vi "DT_Merge_Init.vi"(5 "right subset":cluster{"start idx":i32, "length":i32}, 7 "left subset":cluster{"start idx":i32, "length":i32}, 10 "Triangles In":i32[][](array[numeric]), 11 "Points In":cluster{"x":dbl, "y":dbl, "index":i32}[](array[cluster])) -> (0 "error":i32, 1 "Data":T1, 2 "Triangles Out":i32[][](array[numeric]), 3 "Points Out":cluster{"x":dbl, "y":dbl, "index":i32}[](array[cluster]))   [LabVIEW 2020, in "NI_AAL_Geometry.lvlib"]
uses:
  <vilib>/Analysis/NI_AAL_Geometry.lvlib
  <vilib>/Analysis/geometry.llb/DT_Merge_Find Next Triangulation_Data.ctl
  <vilib>/Analysis/geometry.llb/DT_Triangle Manager_Get Oppo Point_in Ghost.vi
  <vilib>/Analysis/geometry.llb/DT_Triangle Manager_Get Global Point Index.vi
  <vilib>/Analysis/geometry.llb/DT_Triangle Manager_Get Adj_by Edge.vi
  <vilib>/Analysis/geometry.llb/DT_Triangle Manager_Get Oppo Point.vi
  <vilib>/Analysis/geometry.llb/DT_Triangle Manager_Get Ghost Point.vi
  <vilib>/Analysis/geometry.llb/DT_Triangle Manager_Get Adj_by Point.vi
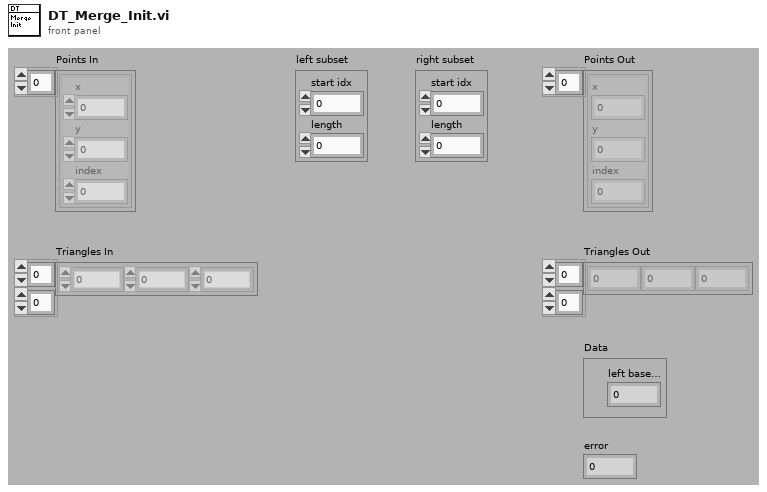
[diagram p1: front panel]
types:
  T1 = typedef "NI_AAL_Geometry.lvlib/DT_Merge_Find Next Triangulation_Data.ctl" = cluster{"left base point":i32, "left triangle":i32, "left local idx":i32, "right base point":i32, "right triangle":i32, "right local idx":i32, "Left Candidate Triangles":i32[], "Left Candidate Point Idx":i32[], "Right Candidate Triangles":i32[], "Right Candidate Point Idx":i32[], "cur triangle":i32}
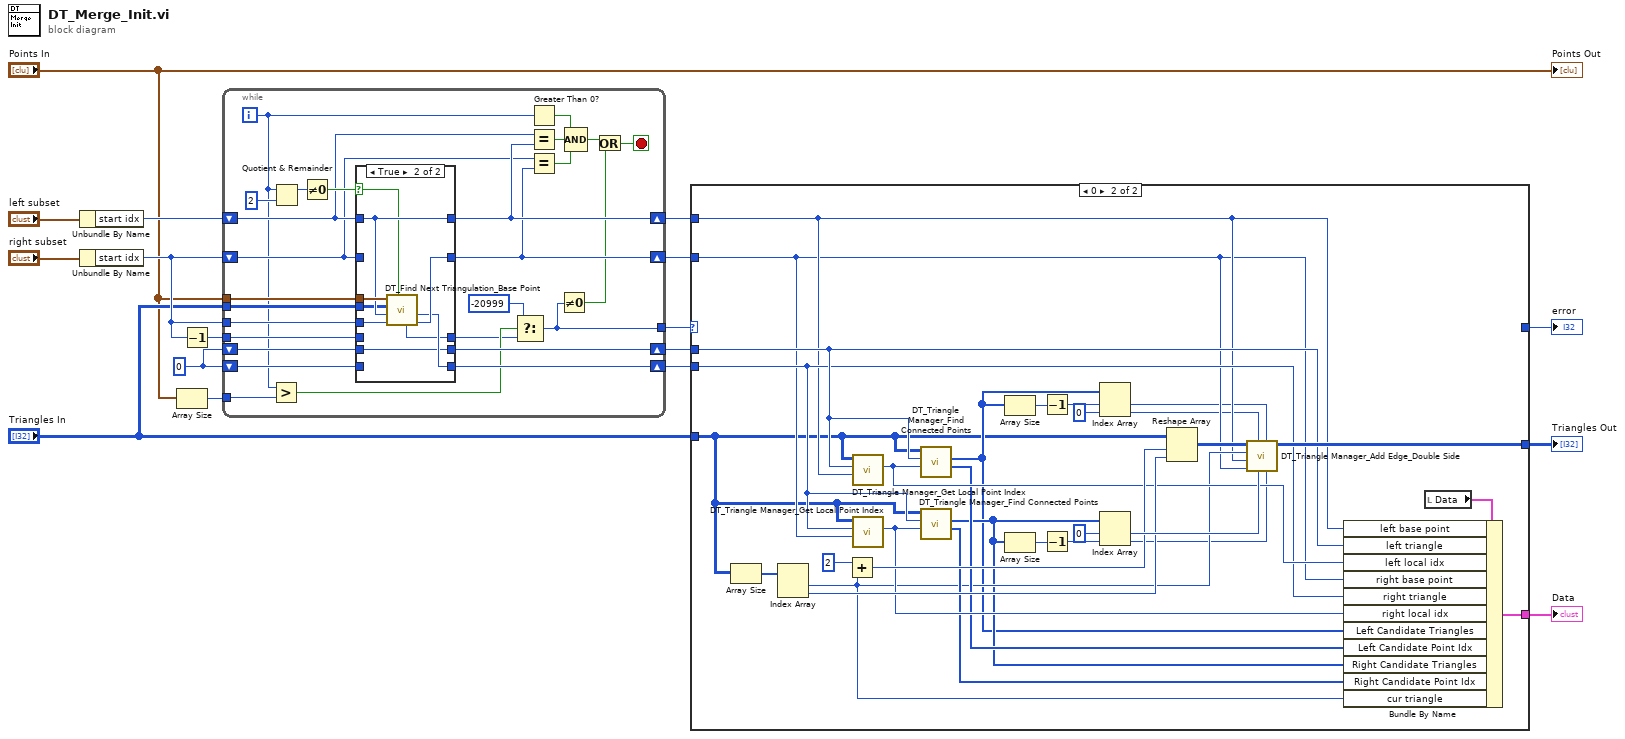
[diagram p0: block diagram]
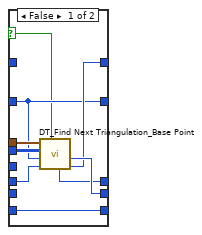
[diagram p3: hidden frame]
diagram:
  w15 = 0 ("triangle")
  n1 = Unbundle By Name("left subset") -> ("start idx"=w7:i32)
  n2 = Unbundle By Name("right subset") -> ("start idx"=w6:i32)
  n3 = Array Size(array="Points In") -> (size(s)=w2:i32)
  n4 = Decrement(x=w6) -> (x-1=w14:i32)
  n5 = while {
    shift-right: [w39] -> w9
    shift-left: w7 -> [w40]
    shift-right: [w37] -> w8
    shift-left: w6 -> [w38]
    shift-right: [w33] -> w11
    shift-left: w15 -> [w31]
    shift-right: [w32] -> w10
    shift-left: w15 -> [w30]
    tunnel: w6 -> [w28]
    tunnel: w14 -> [w29]
    tunnel: "Points In" -> [w44]
    tunnel: "Triangles In" -> [w27]
    tunnel: [w19] -> w4
    tunnel: w2 -> [w22]
    i -> [w23]
    stop <- w24 stop-if-true
    n6 = Greater?(x=w23, y=w22) -> (0:w21:bool)
    n7 = Quotient & Remainder(x=w23, y=2) -> (x-y*floor(x/y)=w42:i32)  [unwired: 1 out]
    n8 = Not Equal To 0?(x=w42) -> (x != 0?=w41:bool)
    n9 = case shown="True" w41 {
      selector: w41 -> [w46 w55]
      tunnel: w44 -> [w53 w62]
      tunnel: w27 -> [w52 w57]
      tunnel: w40 -> [_ w60]
      tunnel: w38 -> [w49 _]
      tunnel: [w49 w61] -> w37
      tunnel: [w50 w60] -> w39
      tunnel: [w51 w58] -> w33
      tunnel: [w48 w59] -> w32
      tunnel: w31 -> [_ w58]
      tunnel: w30 -> [w48 _]
      tunnel: w29 -> [w47 _]
      tunnel: w28 -> [_ w56]
      tunnel: [w45 w54] -> w20
      frame False {
        n10 = call <vilib>:"DT_Find Next Triangulation_Base Point.vi"("left/right pt (right:F)"=w46, "search point"=w47, "external point"=w49, "Triangles In"=w52, "Points In"=w53) -> ("base point"=w50:i32, "triangle"=w51:i32, "error"=w45:i32)  [unwired: 1 in, 3 out]
      }
      frame True {
        n11 = call <vilib>:"DT_Find Next Triangulation_Base Point.vi"("left/right pt (right:F)"=w55, "search point"=w56, "external point"=w60, "Triangles In"=w57, "Points In"=w62) -> ("base point"=w61:i32, "triangle"=w59:i32, "error"=w54:i32)  [unwired: 1 in, 3 out]
      }
    }
    n12 = Select(t=-20999, s=w21, f=w20) -> (s? t:f=w19:i32)
    n13 = Greater Than 0?(x=w23) -> (x > 0?=w36:bool)
    n14 = Equal?(x=w40, y=w39) -> (x = y?=w35:bool)
    n15 = Equal?(x=w38, y=w37) -> (x = y?=w34:bool)
    n16 = Not Equal To 0?(x=w19) -> (x != 0?=w25:bool)
    n17 = Compound Arithmetic op=AND(w36, w35, w34) -> (w26:bool)
    n18 = Or(x=w26, y=w25) -> (x .or. y?=w24:bool)
  }
  n19 = case shown="0" w4 {
    selector: w4 -> [w63 _]
    tunnel: [_ w92] -> w13
    tunnel: [_ w86] -> w12
    tunnel: w11 -> [_ w85]
    tunnel: w10 -> [_ w83]
    tunnel: w9 -> [_ w78]
    tunnel: w8 -> [_ w77]
    tunnel: "Triangles In" -> [_ w64]
    tunnel: [w63 _] -> w5
    frame Default {
    }
    frame 0 {
      n20 = Array Size(array=w64) -> (size(s)=w91:i32[])
      n21 = Index Array(array=w91) -> (element #1=w79:i32, element #2=w89:i32)  [unwired: 2 in]
      n22 = Add(x=2, y=w79) -> (x+y=w87:i32)
      n23 = call <vilib>:"DT_Triangle Manager_Get Local Point Index.vi"("global idx"=w78, "triangle"=w85, "Triangles"=w64) -> ("local idx"=w84:i32)  [unwired: 8 out]
      n24 = call <vilib>:"DT_Triangle Manager_Get Local Point Index.vi"("global idx"=w77, "triangle"=w83, "Triangles"=w64) -> ("local idx"=w82:i32)  [unwired: 8 out]
      n25 = call <vilib>:"DT_Triangle Manager_Find Connected Points.vi"("base point idx"=w84, "triangle"=w85, "Triangles"=w64) -> ("Connected Point Idx"=w81:i32[], "Connected Triangles"=w70:i32[])  [unwired: 7 out]
      n26 = call <vilib>:"DT_Triangle Manager_Find Connected Points.vi"("base point idx"=w82, "triangle"=w83, "Triangles"=w64) -> ("Connected Point Idx"=w80:i32[], "Connected Triangles"=w75:i32[])  [unwired: 7 out]
      n27 = Array Size(array=w70) -> (size(s)=w71:i32)
      n28 = Array Size(array=w75) -> (size(s)=w76:i32)
      n29 = Decrement(x=w71) -> (x-1=w69:i32)
      n30 = Decrement(x=w76) -> (x-1=w74:i32)
      n31 = Index Array(array=w70, index #1=w69, index #2=0 ("index")) -> (element #1=w67:i32, element #2=w66:i32)
      n32 = Index Array(array=w75, index #1=0 ("index"), index #2=w74) -> (element #1=w93:i32, element #2=w73:i32)
      n33 = Reshape Array(w64, w87, w89) -> (w90:i32[][])
      n34 = call <vilib>:"DT_Triangle Manager_Add Edge_Double Side.vi"("right bottom tri"=w73, "left bottom tri"=w67, "right top tri"=w93, "left top tri"=w66, "right point"=w77, "left point"=w78, "next triangle in"=w79, "Triangles In"=w90) -> ("Triangles Out"=w92:i32[][])  [unwired: 3 out]
      n35 = local read "Data"() -> (w65:T1)
      n36 = Bundle By Name(cluster=w65, "left base point"=w78, "left triangle"=w85, "left local idx"=w84, "right base point"=w77, "right triangle"=w83, "right local idx"=w82, "Left Candidate Triangles"=w70, "Left Candidate Point Idx"=w81, "Right Candidate Triangles"=w75, "Right Candidate Point Idx"=w80, "cur triangle"=w79) -> (w86:T1)
    }
  }
  "Triangles Out" <- w13
  "Data" <- w12
  "error" <- w5
  "Points Out" <- "Points In"
